vi "onIncomingMessagingError.vi"(8 "error in (no error)":errorcluster, 10 "model in":refnum<class "IModel.lvclass">, 11 "EnabledState in":refnum<class "EnabledState.lvclass">) -> (0 "error out":errorcluster, 2 "model out":refnum<class "IModel.lvclass">, 3 "EnabledState out":refnum<class "EnabledState.lvclass">)   [LabVIEW 2016, in "States.lvlib" / "EnabledState.lvclass"]
uses:
  EnabledState.lvclass
  IModel/IModel.lvclass
  Typedefs/StateValue.ctl
  ts_sallv_exa/DataTypes/logevent_SummaryState.ctl
  ComponentTemplateCore/ComponentModel/ComponentModel/InternalSignals/error.vi
  Typedefs/EXATypedefs.lvlib
  ComponentTemplateCore/ComponentModel/ComponentModel/InternalSignals/InternalSignalsGlobals.lvlib
  ts_sallv_exa/SALLV_EXA.lvlib
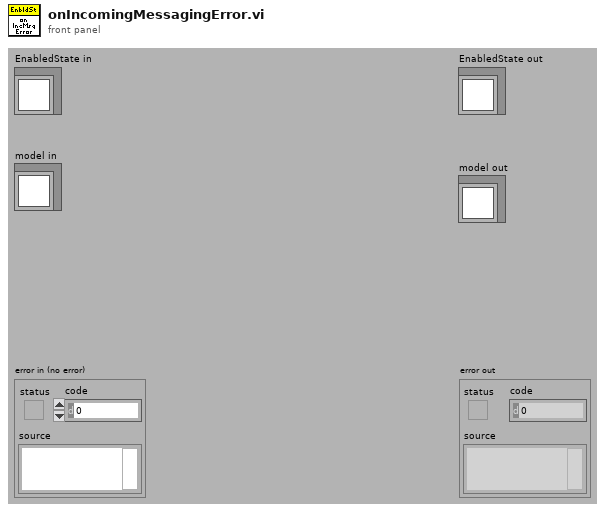
[diagram p1: front panel]
types:
  T1 = typedef "SALLV_EXA.lvlib/logevent_SummaryState.ctl" = cluster{"summaryState":enum16{"", " OfflineState", "StandbyState", "DisabledState", "EnabledState", "FaultState"}, "priority":i32}
  T2 = typedef "EXATypedefs.lvlib/StateValue.ctl" = enum16{"OffState", "StandbyState", "DisabledState", "EnabledState", "FaultState"}
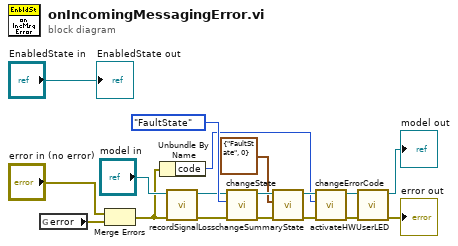
[diagram p0: block diagram]
diagram:
  n1 = global read "error.vi" "error"() -> (w10:errorcluster)
  n2 = Merge Errors("error in (no error)", w10) -> (w3:errorcluster)
  n3 = Unbundle By Name(w3) -> ("code"=w11:i32)
  n4 = call-dynamic "recordSignalLoss.vi"("error in (no error)"=w3, "IModel in"="model in") -> ("error out"=w2:errorcluster, "IModel out"=w4:refnum<class "IModel.lvclass">)  [unwired: 8 in]
  n5 = call-dynamic "changeState.vi"("error in (no error)"=w2, "newState"=StateValue."FaultState" ("DetailedStateValue"), "IModel in"=w4) -> ("error out"=w13:errorcluster, "IModel out"=w15:refnum<class "IModel.lvclass">)  [unwired: 7 in]
  n6 = call-dynamic "changeSummaryState.vi"("error in (no error)"=w13, "logevent_SummaryState"=T1 {"summaryState"=enum."FaultState", "priority"=0}, "IModel in"=w15) -> ("error out"=w12:errorcluster, "IModel out"=w14:refnum<class "IModel.lvclass">)  [unwired: 7 in]
  n7 = call-dynamic "changeErrorCode.vi"("error in (no error)"=w12, "error.code"=w11, "IModel in"=w14) -> ("error out"=w7:errorcluster, "IModel out"=w9:refnum<class "IModel.lvclass">)  [unwired: 7 in]
  n8 = call-dynamic "activateHWUserLED.vi"("error in (no error)"=w7, "IModel in"=w9) -> ("error out"=→"error out":errorcluster, "IModel out"=→"model out":refnum<class "IModel.lvclass">)  [unwired: 8 in]
  "EnabledState out" <- "EnabledState in"
